vi "DroneMeasureAngle.vi"() -> ()   [LabVIEW 2017]
uses:
  <vilib>/LVH/AR Drone Toolkit/Decode NavData/Typedefs/NavData Demo.ctl
  <vilib>/LVH/AR Drone Toolkit/AR Drone.lvlib
panel:
  in  "Measure":bool
  in  "Setup Parameters":T1={"Drone IP address"="192.168.1.1", "Home IP address"="192.168.1.2", "Flight Mode"=enum."INDOOR MODE", "Mounted Hull"=enum."INDOOR HULL", "Video Camera"=2, "Max Altitude (m)"=3.0, "Max Pitch and Roll Angle (deg)"=10.0, "Max Vertical Speed (m/s)"=0.7, "Max Yaw Speed (deg/s)"=100.0} {"Video Camera" items=["Bottom Camera"=1, "Front Camera"=0, "Front in Bottom"=3, "Bottom in Front"=2]}
  out "Caliper Results (Caliper 1)":sgl[][](array[numeric]) format="%.2f"
  out "Video Stream":picture
  out "NavData Out":T2
  out "Battery Remaining":dbl(slide) scale=0.0..100.0
  in  "Hover":bool
  in  "Take Off/Land":bool
  in  "Emergency Landing":bool
  in  "stop 2":bool
  in  "Control Cluster":T3 {"Yaw Speed" scale=-1.0..1.0; "Vertical Speed" scale=-1.0..1.0; "Pitch" scale=-1.0..1.0; "Roll" scale=-1.0..1.0}
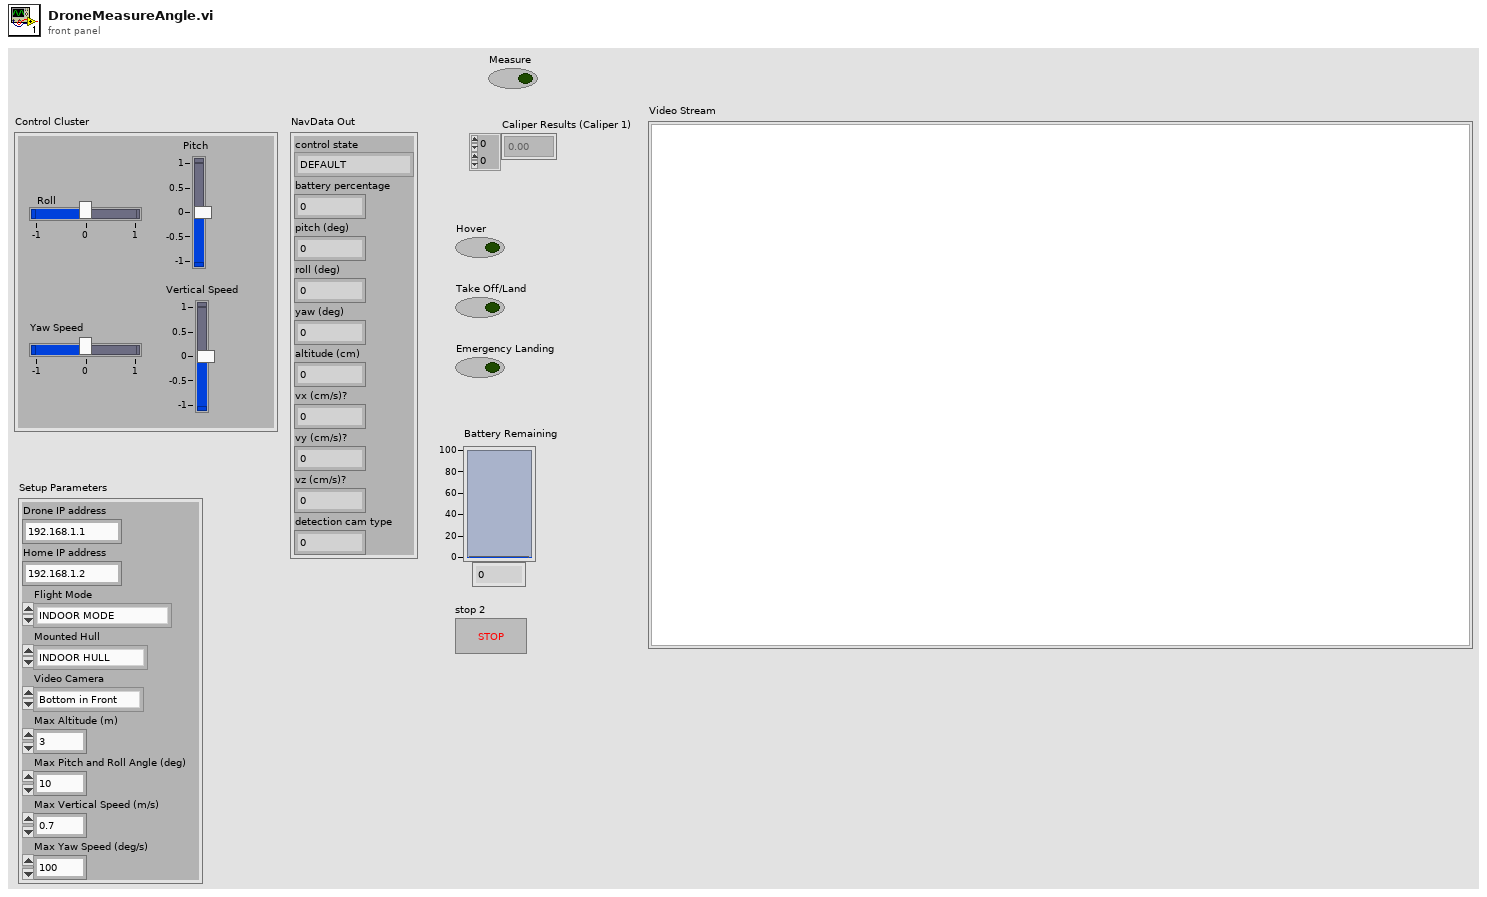
[diagram p1: front panel]
types:
  T1 = cluster{"Drone IP address":string, "Home IP address":string, "Flight Mode":enum8{"OUTDOOR MODE", "INDOOR MODE"}, "Mounted Hull":enum8{"OUTDOOR HULL", "INDOOR HULL"}, "Video Camera":u8, "Max Altitude (m)":sgl, "Max Pitch and Roll Angle (deg)":sgl, "Max Vertical Speed (m/s)":sgl, "Max Yaw Speed (deg/s)":sgl}
  T2 = typedef "AR Drone.lvlib/NavData Demo.ctl" = cluster{"control state":enum32{"DEFAULT", "INIT", "LANDING", "FLYING", "HOVERING", "TEST", "TRANS_TAKEOFF", "TRANS_GOTOFIX", "TRANS_LANDING"}, "battery percentage":u32, "pitch (deg)":sgl, "roll (deg)":sgl, "yaw (deg)":sgl, "altitude (cm)":u32, "vx (cm/s)?":sgl, "vy (cm/s)?":sgl, "vz (cm/s)?":sgl, "detection cam type":u32}
  T3 = cluster{"Roll":sgl, "Pitch":sgl, "Vertical Speed":sgl, "Yaw Speed":sgl}
  T4 = typedef "AR Drone.lvlib/AR Drone Resource.ctl" = cluster{"UDP Control Connection":refnum<k16>, "UDP NavData Connection":refnum<k16>, "UDP Video Connection (Drone 1.0)":refnum<k16>, "TCP Video Connection (Drone 2.0)":refnum<k5>, "TCP Control Port Connection":refnum<k5>, "Drone IP address":string, "Drone Command Port":u16, "Drone NavData Port":u16, "Drone Vid Stream Port":u16, "Drone TCP Control Port":u16, "Home IP address":string, "Home Command Port":u16, "Home NavData Port":u16, "Home Vid Stream Port":u16, "Drone Version":i32, "Drone Index":dbl}
  T5 = typedef "IMAQ Image.ctl" = refnum<image>
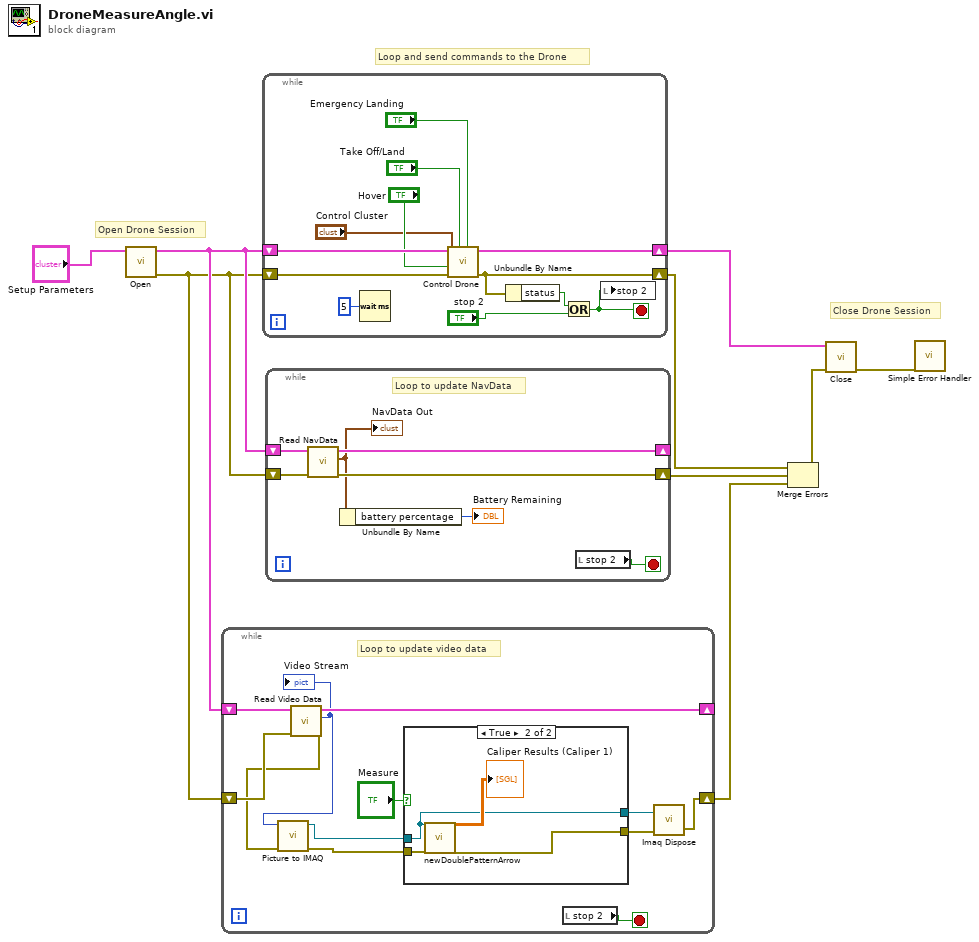
[diagram p0: block diagram]
diagram:
  # "Close Drone Session"
  # "Loop and send commands to the Drone"
  # "Open Drone Session"
  n1 = call <vilib>:"Open.vi"("Setup Parameters"="Setup Parameters") -> ("error out"=w6:errorcluster, "AR Drone Resource"=w7:T4)  [unwired: 9 in]
  n2 = while {
    shift-right: [w18] -> _
    shift-left: w7 -> [w20]
    shift-right: [w10] -> w1
    shift-left: w6 -> [w19]
    stop <- w21 stop-if-true
    # "Loop to update video data"
    n3 = call <vilib>:"Read Video Data.vi"("error in (no error)"=w19, "AR Drone Resource"=w20) -> ("error out"=w17:errorcluster, "Video Stream"=w16:picture, "AR Drone Resource Out"=w18:T4)  [unwired: 7 in]
    "Video Stream" <- w16
    n4 = call "Picture to IMAQ.vi"("Error In"=w17, "picture"=w16) -> ("Error Out"=w14:errorcluster, "Image"=w15:T5)  [unwired: 8 in]
    n5 = case shown="True" "Measure" {
      tunnel: w15 -> [w22 w24]
      tunnel: w14 -> [w23 w27]
      tunnel: [w23 w26] -> w13
      tunnel: [w22 w24] -> w12
      frame False {
      }
      frame True {
        n6 = call "newDoublePatternArrow.vi"("Image In"=w24, "error in (no error)"=w27) -> ("Caliper Results (Caliper 1)"=→"Caliper Results (Caliper 1)":sgl[][], "error out"=w26:errorcluster)  [unwired: 24 in]
      }
    }
    n7 = local read "stop 2"() -> (w21:bool)
    n8 = call "Imaq Dispose"("Image"=w12, "error in (no error)"=w13) -> ("error out"=w10:errorcluster)  [unwired: 4 in]
  }
  n9 = while {
    shift-right: [w34] -> w9
    shift-left: w7 -> [w38]
    shift-right: [w29] -> w3
    shift-left: w6 -> [w39]
    stop <- w28 stop-if-true
    n10 = Wait (ms)(milliseconds to wait=u32 5) -> ()  [unwired: 1 out]
    n11 = call <vilib>:"Control Drone.vi"("Emergency Landing"="Emergency Landing", "Takeoff/Land"="Take Off/Land", "error in (no error)"=w39, "Hover"="Hover", "Control Cluster"="Control Cluster", "AR Drone Resource"=w38) -> ("error out"=w29:errorcluster, "AR Drone Resource Out"=w34:T4)  [unwired: 4 in]
    n12 = Unbundle By Name(w29) -> ("status"=w31:bool)
    n13 = Or(x=w31, y="stop 2") -> (x .or. y?=w28:bool)
    n14 = local write "stop 2"(w28) -> ()
  }
  n15 = while {
    shift-right: [w44] -> _
    shift-left: w7 -> [w45]
    shift-right: [w42] -> w4
    shift-left: w6 -> [w43]
    stop <- w46 stop-if-true
    # "Loop to update NavData"
    n16 = call <vilib>:"Read NavData.vi"("error in (no error)"=w43, "AR Drone Resource"=w45) -> ("error out"=w42:errorcluster, "NavData Out"=w41:T2, "AR Drone Resource Out"=w44:T4)  [unwired: 7 in]
    "NavData Out" <- w41
    n17 = Unbundle By Name(w41) -> ("battery percentage"=→"Battery Remaining":u32)
    n18 = local read "stop 2"() -> (w46:bool)
  }
  n19 = Merge Errors(w3, w4, w1) -> (w5:errorcluster)
  n20 = call <vilib>:"Close.vi"("error in (no error)"=w5, "AR Drone Resource"=w9) -> ("error out"=w8:errorcluster)  [unwired: 9 in]
  n21 = call <vilib>:"Simple Error Handler.vi"("error in (no error)"=w8) -> ()  [unwired: 4 in, 5 out]
